vi "Get Scanner.vi"(8 "error in (no error)":errorcluster, 11 "Magna Power in":refnum<class "Magna Power.lvclass">) -> (0 "error out":errorcluster, 2 "Default Scanner out":refnum<class "Scanner.lvclass">)   [LabVIEW 2012, in "Magna Power.lvclass"]
doc: "(Dynamic) Returns the default Scanner object that scans over this Scannable. (Note that a Scannable may have multiple Scanners associated with it.) A Scanner is an analogue to an Iterator class in other languages."
uses:
  Magna Power.lvclass
  Scanners/Scanner/Scanner.lvclass
  Utility Classes/Scannable/Scannable.lvclass
  Scanners/Magna Power Scan/Magna Power Scan.lvclass
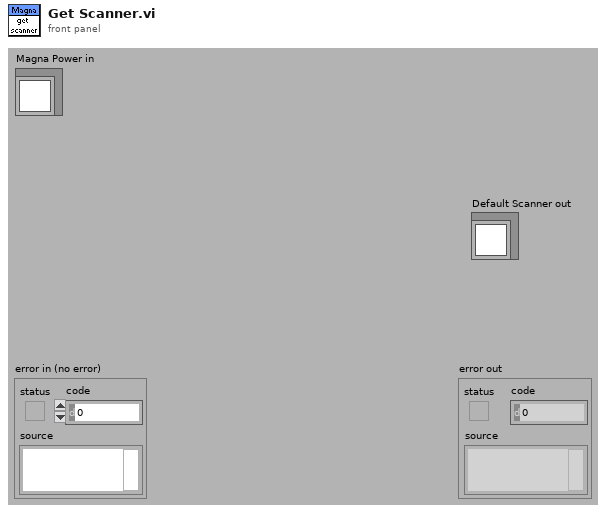
[diagram p1: front panel]
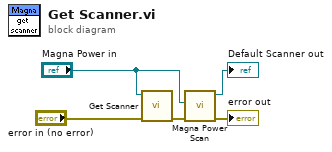
[diagram p0: block diagram]
diagram:
  n1 = call-parent "Get Scanner.vi"("error in (no error)"="error in (no error)", "Scannable in"="Magna Power in") -> ("error out"=w4:errorcluster)  [unwired: 8 in, 1 out]
  n2 = call "Magna Power Scan.vi"("error in (no error)"=w4, "Magna Power.lvclass"="Magna Power in") -> ("error out"=→"error out":errorcluster, "Magna Power Scan.lvclass out"=→"Default Scanner out":refnum<class "Magna Power Scan.lvclass">)  [unwired: 8 in]
